vi "Scorer Post.vi"(8 "error in (no error)":errorcluster, 10 "buffer":string, 11 "Path":string="/scoring/next") -> (0 "error out":errorcluster, 2 "Status":i32, 3 "Content":string, 5 "Profile URL":string)   [LabVIEW 2024, in "Wordle Scorer.lvlib"]
uses:
  Wordle Scorer.lvlib
  <vilib>/httpClient/LabVIEWHTTPClient.lvlib
  <vilib>/httpClient/POSTBuffer.vi
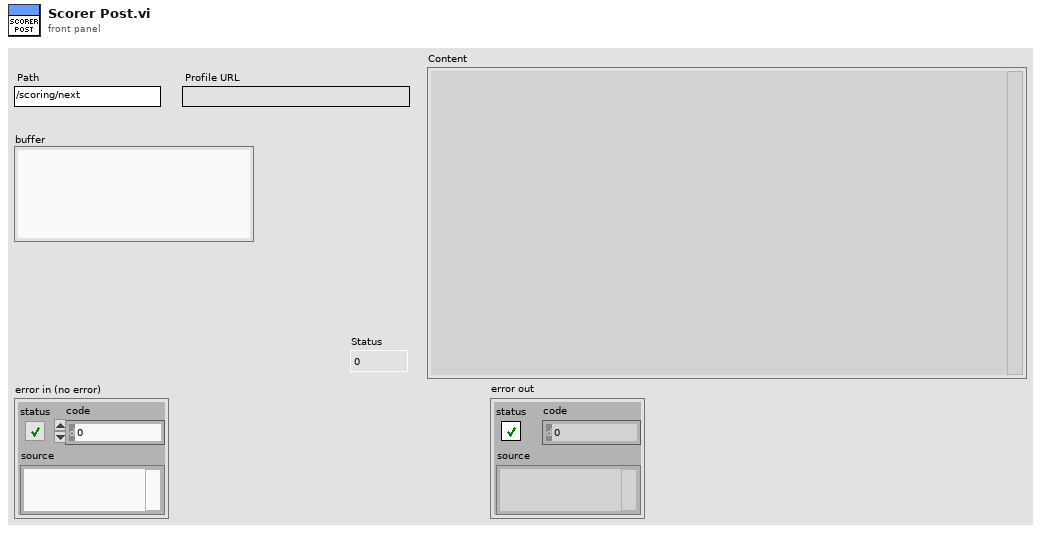
[diagram p1: front panel]
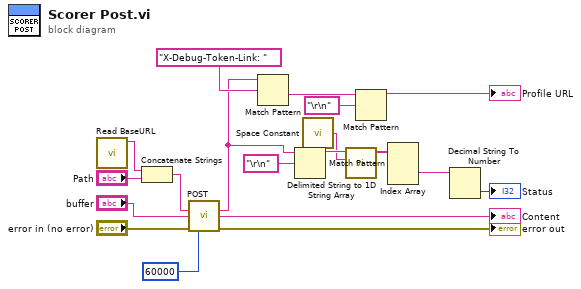
[diagram p0: block diagram]
diagram:
  n1 = call "Read BaseURL.vi"() -> ("BaseURL"=w12:string)  [unwired: 10 in, 1 out]
  n2 = Concatenate Strings(w12, "Path") -> (w18:string)
  n3 = call-poly <vilib>:"POST.vi"("url"=w18, "buffer"="buffer", "error in (no error)"="error in (no error)", "timeout (10000)"=60000) -> ("headers"=w10:string, "body"=→"Content":string, "error out"=→"error out":errorcluster)  [unwired: 8 in, 1 out]
  n4 = Match Pattern(string=w10, regular expression="X-Debug-Token-Link: ") -> (after substring=w15:string)  [unwired: 1 in, 3 out]
  n5 = Match Pattern(string=w10, regular expression="\r\n") -> (before substring=w9:string)  [unwired: 1 in, 3 out]
  n6 = call <vilib>:"Space Constant.vi"() -> ("String"=w8:string)
  n7 = call <vilib>:"Delimited String to 1D String Array.vi"("delimiter"=w8, "delimited string"=w9) -> ("string array"=w7:string[])  [unwired: 9 in]
  n8 = Match Pattern(string=w15, regular expression="\r\n") -> (before substring=→"Profile URL":string)  [unwired: 1 in, 3 out]
  n9 = Index Array(array=w7) -> (element #2=w6:string)  [unwired: 3 in, 2 out]
  n10 = Decimal String To Number(string=w6) -> (number=→"Status":i32)  [unwired: 2 in, 1 out]
